vi "1WIRE_Write_Byte_multi.vi"(8 "error in":errorcluster, 10 "Tx data":u8, 11 "FPGA I/O":refnum<k21>="DS_WIRE") -> (0 "error out":errorcluster, 2 "Written":bool[](array[boolean]))   [LabVIEW 2014]
doc: "This VI is created by Vincent Claes for FPDA-1 more information on http://pwo.fpga.be\n\nvincent.claes@xios.be\nclaesvincent@gmail.com\n\nhttp://www.linkedin.com/in/vincentclaes"
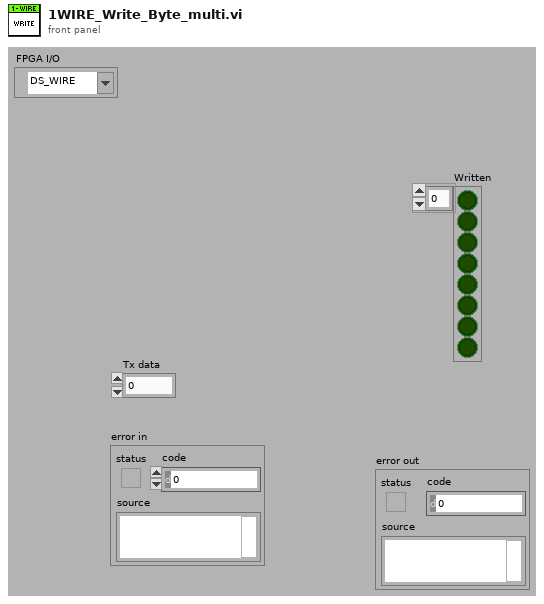
[diagram p1: front panel]
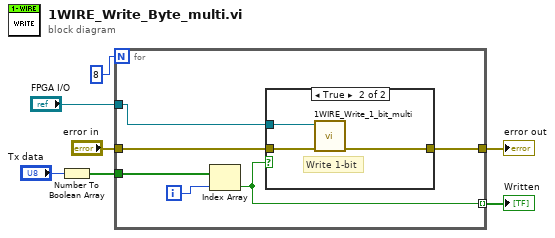
[diagram p0: block diagram]
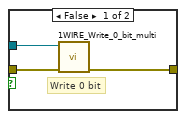
[diagram p2: hidden frame]
diagram:
  n1 = Number To Boolean Array(number="Tx data") -> (Boolean array=w7:bool[])
  n2 = for {
    N: 8 -> [_]
    tunnel: w7 -> [w13]
    tunnel: [w12] -> w4
    tunnel: "error in" -> [w11]
    tunnel: [w9] -> w2 mode=indexing
    tunnel: "FPGA I/O" -> [w8]
    i -> [w10]
    n3 = Index Array(array=w13, index=w10) -> (element=w9:bool)
    n4 = case shown="True" w9 {
      tunnel: [w15 w18] -> w12
      tunnel: w11 -> [w16 w19]
      tunnel: w8 -> [w14 w17]
      frame False {
        # "Write 0 bit"
        n5 = call "1WIRE_Write_0_bit_multi.vi"("error in"=w16, "FPGA I/O"=w14) -> ("error out"=w15:errorcluster)  [unwired: 9 in]
      }
      frame True {
        # "Write 1-bit"
        n6 = call "1WIRE_Write_1_bit_multi.vi"("error in"=w19, "FPGA I/O"=w17) -> ("error out"=w18:errorcluster)  [unwired: 9 in]
      }
    }
  }
  "error out" <- w4
  "Written" <- w2
